vi "CustomRunTimeMenu.vi"(3 "Menu Items":T1(array[cluster]), 4 "Global Menu Refnum Set":refnum<k4>, 5 "Menu Ready Occurrance":refnum<k4>) -> (0 "error out":errorcluster, 1 "MenuItemNames":string[](array[string]))   [LabVIEW 2012]
uses:
  GlobalMenuReference.vi
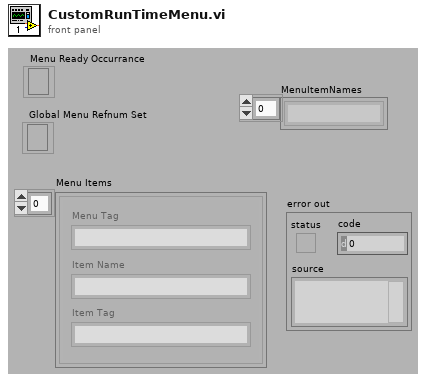
[diagram p1: front panel]
types:
  T1 = cluster{"Menu Tag":string, "Item Name":string, "Item Tag":string}[]
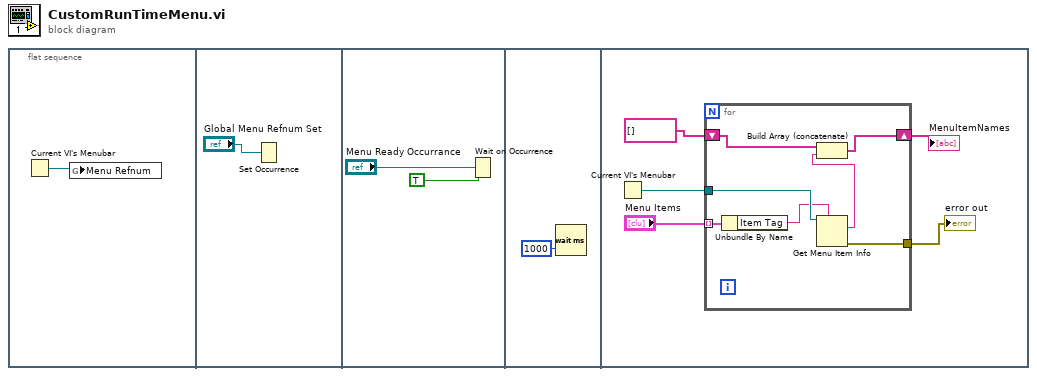
[diagram p0: block diagram]
diagram:
  n1 = flat-sequence {
    frame #0 {
      n2 = Current VI's Menubar() -> (w1:refnum<k9>)
      n3 = global write "GlobalMenuReference.vi" "Menu Refnum"(w1) -> ()
    }
    frame #1 {
      n4 = Set Occurrence("Global Menu Refnum Set") -> ()
    }
    frame #2 {
      n5 = Wait on Occurrence(1:TRUE ("ignore previous (T)"), 2:"Menu Ready Occurrance") -> ()  [unwired: 2 out]
    }
    frame #3 {
      n6 = Wait (ms)(milliseconds to wait=u32 1000) -> ()  [unwired: 1 out]
    }
    frame #4 {
      n7 = Current VI's Menubar() -> (w9:refnum<k9>)
      n8 = for {
        tunnel: "Menu Items" -> [w17] mode=indexing
        tunnel: w9 -> [w16]
        shift-right: [w12] -> w7
        shift-left: string[] [] -> [w14]
        tunnel: [w11] -> w6
        n9 = Unbundle By Name(w17) -> ("Item Tag"=w15:string)
        n10 = Get Menu Item Info(7:w15, 11:w16) -> (0:w11:errorcluster, 2:w13:string)  [unwired: 1 in, 5 out]
        n11 = Build Array (concatenate)(w14, w13) -> (w12:string[])
      }
      "MenuItemNames" <- w7
      "error out" <- w6
    }
  }
